vi "Update status display-Z plane.vi"(8 "error in (no error)":errorcluster, 9 "Imaging Protocol":T1, 10 "Acquired z-plane index":i32, 11 "Message Queues":T2) -> (0 "error out":errorcluster)   [LabVIEW 2013]
uses:
  Queue/Message Queue/Typedefs/All Message Queues.ctl
  Queue/Message Queue/Typedefs/Message Cluster.ctl
  Typedefs/Logging queue element.ctl
  Typedefs/Imaging Protocols enum.ctl
  Typedefs/Frame Size.ctl
  Typedefs/Acquired points count.ctl
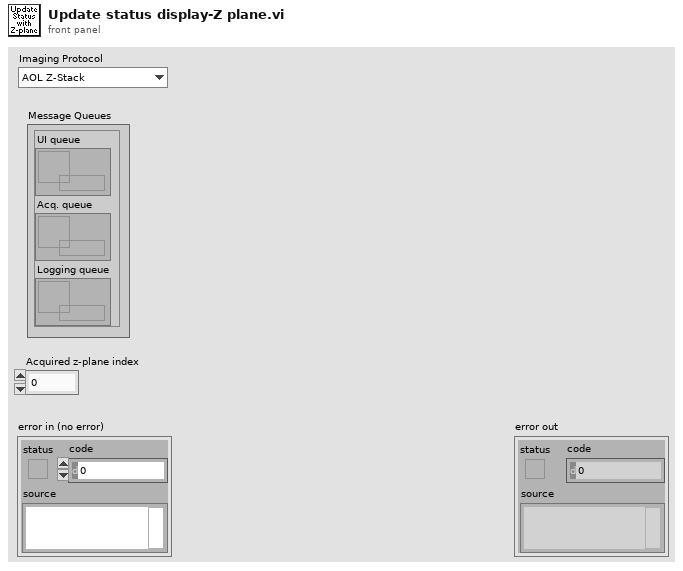
[diagram p1: front panel]
types:
  T1 = typedef "Imaging Protocols enum.ctl" = enum16{"AOL Z-Stack", "Motor Z Stack", "Functional Acquisition", "Single Plane Acquisition", "Volume Acquisition", "Live Imaging", "Live Plane Imaging", "Live Volume Imaging"}
  T2 = typedef "All Message Queues.ctl" = cluster{"UI queue":refnum<queue>, "Acq. queue":refnum<queue>, "Logging queue":refnum<queue>}
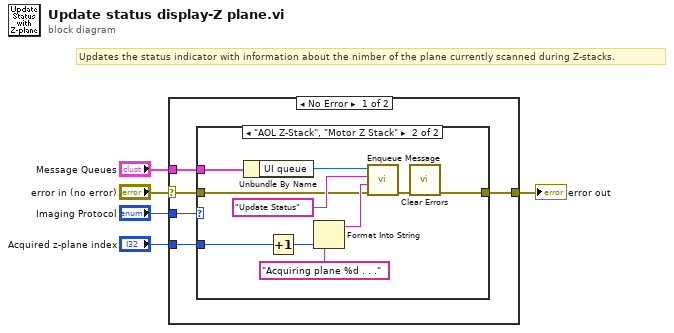
[diagram p0: block diagram]
diagram:
  # "Updates the status indicator with information about the nimber of the plane currently scanned during Z-stacks."
  n1 = case shown="No Error" "error in (no error)" {
    selector: "error in (no error)" -> [w6 w22]
    tunnel: "Acquired z-plane index" -> [w10 _]
    tunnel: "Message Queues" -> [w9 _]
    tunnel: "Imaging Protocol" -> [w7 _]
    tunnel: [w8 w22] -> w1
    frame No Error {
      n2 = case shown="\"AOL Z-Stack\", \"Motor Z Stack\"" w7 {
        tunnel: w10 -> [_ w17]
        tunnel: w9 -> [_ w16]
        tunnel: [w11 w15] -> w8
        tunnel: w6 -> [w11 w12]
        frame Default {
        }
        frame "AOL Z-Stack", "Motor Z Stack" {
          n3 = Unbundle By Name(w16) -> ("UI queue"=w19:refnum<queue>)
          n4 = Increment(x=w17) -> (x+1=w13:i32)
          n5 = Format Into String(format string="Acquiring plane %d . . .", w13) -> (resulting string=w21:string)  [unwired: 2 in, 1 out]
          n6 = call "Enqueue Message.vi"("error in (no error)"=w12, "Message Data"=w21, "Message"="Update Status", "Queue"=w19) -> ("error out"=w20:errorcluster)  [unwired: 6 in, 1 out]
          n7 = call <vilib>:"Clear Errors.vi"("error in (no error)"=w20) -> ("error out"=w15:errorcluster)  [unwired: 6 in]
        }
      }
    }
    frame Error {
    }
  }
  "error out" <- w1
